vi "Switch From Symbol.vi"(9 "Level Items":T1[](array[typedef]), 11 "On Symbol":i32) -> (2 "Array":bool[](array[boolean]))   [LabVIEW 2024]
uses:
  Ancestor Class/Front Panel Container/Tree/Tree/Type Def/Tree Item.ctl
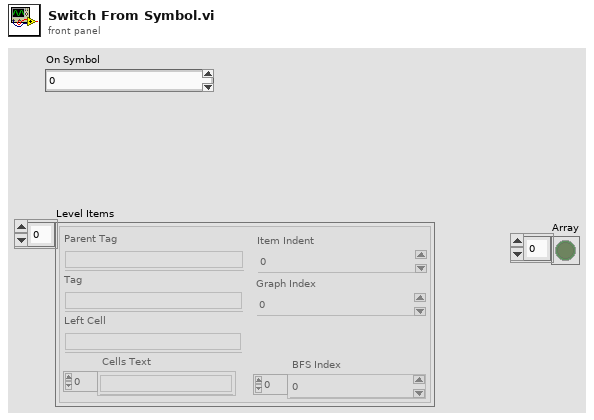
[diagram p1: front panel]
types:
  T1 = typedef "Tree Item.ctl" = cluster{"Parent Tag":string, "Tag":string, "Left Cell":string, "Cells Text":string[], "BFS Index":i32[], "Graph Index":i32, "Item Indent":i32}
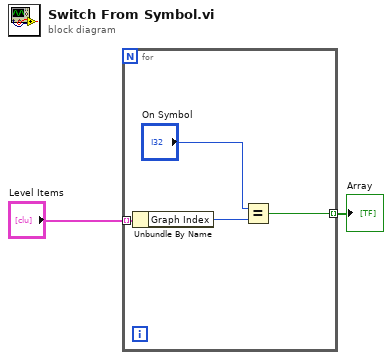
[diagram p0: block diagram]
diagram:
  n1 = for {
    tunnel: "Level Items" -> [w6] mode=indexing
    tunnel: [w3] -> w1 mode=indexing
    n2 = Unbundle By Name(w6) -> ("Graph Index"=w5:i32)
    n3 = Equal?(x="On Symbol", y=w5) -> (x = y?=w3:bool)
  }
  "Array" <- w1
